vi "test.vi"   [LabVIEW 2023]
uses:
  Parent/Parent.lvclass
  Class 1/Class 1.lvclass
  Class 2/Class 2.lvclass
  Class 3/Class 3.lvclass
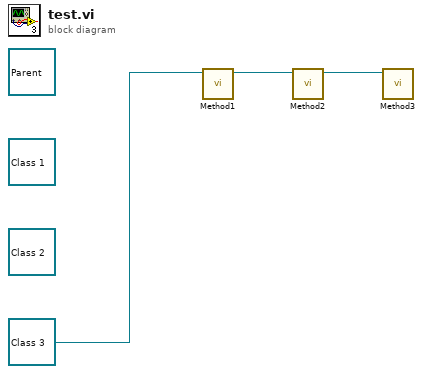
[diagram p0: block diagram]
diagram:
  (unwired) refnum<class "Class 2.lvclass"> refnum ("Class 2.lvclass")
  (unwired) refnum<class "Class 1.lvclass"> refnum ("Class 1.lvclass")
  (unwired) refnum<class "Parent.lvclass"> refnum ("Parent.lvclass")
  n1 = call-dynamic "Method1.vi"("Class 3 in"=refnum<class "Class 3.lvclass"> refnum ("Class 3.lvclass")) -> ("Class 3 out"=w3:refnum<class "Class 3.lvclass">)  [unwired: 9 in, 1 out]
  n2 = call-dynamic "Method2.vi"("Class 3 in"=w3) -> ("Class 3 out"=w2:refnum<class "Class 3.lvclass">)  [unwired: 9 in, 1 out]
  n3 = call-dynamic "Method3.vi"("Class 3 in"=w2) -> ()  [unwired: 9 in, 2 out]
